vi "update table.vi"(5 "Sort By...":T4 items=["RIO device", "resource", "input type", "datatype", "reserver"], 8 "error in (no error)":errorcluster, 10 "MulticolumnListbox in":refnum<vi>, 11 "Item Ref in":T1 format="%.0x") -> (0 "error out":errorcluster, 2 "max string length in columns":i32[](array[numeric]), 3 "fpga resources out":cluster{"fpga cd":T1, "resource":T2}[](array[cluster]) {"fpga cd" format="%.0x"})   [LabVIEW 2016, in "FPGA RM System Definition API.lvlib"]
uses:
  FPGA RM System Definition API.lvlib
  type defs/viz_type.ctl
  <vilib>/NI Veristand/Custom Device API/Custom Device Item Ref.ctl
  Shared/Types/fpga resource.ctl
  Shared/Types/Channel Type.ctl
  UI/visualizer globals.vi
  <vilib>/NI VeriStand/Custom Device API/Custom Device API.lvlib
  Shared/FPGA RM Shared API.lvlib
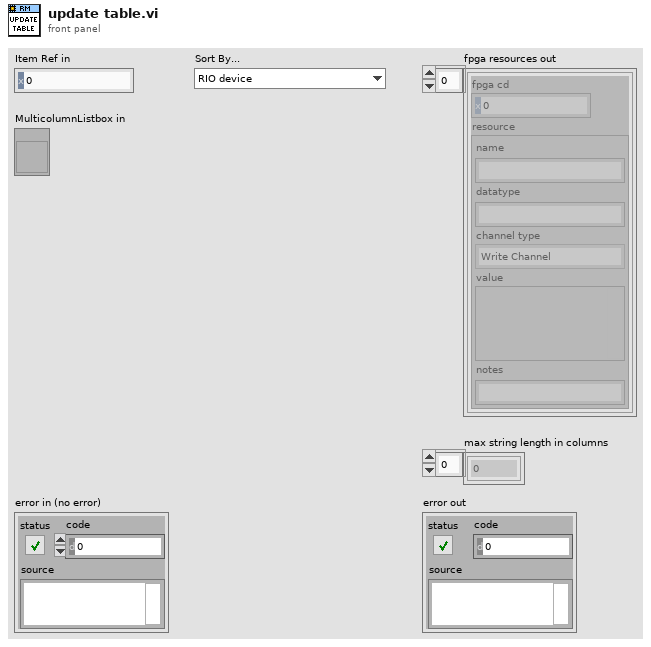
[diagram p1: front panel]
types:
  T1 = typedef "Custom Device API.lvlib/Custom Device Item Ref.ctl" = u64
  T2 = typedef "FPGA RM Shared API.lvlib/fpga resource.ctl" = cluster{"name":string, "datatype":string, "channel type":T3, "value":variant, "notes":string}
  T3 = typedef "FPGA RM Shared API.lvlib/Channel Type.ctl" = enum16{"Write Channel", "Read Channel", "Write Waveform", "Read Waveform"}
  T4 = typedef "FPGA RM System Definition API.lvlib/viz_type.ctl" = u16
  T5 = typedef "FPGA RM System Definition API.lvlib/resources.ctl" = cluster{"fpga cd":T1, "resource":T2}
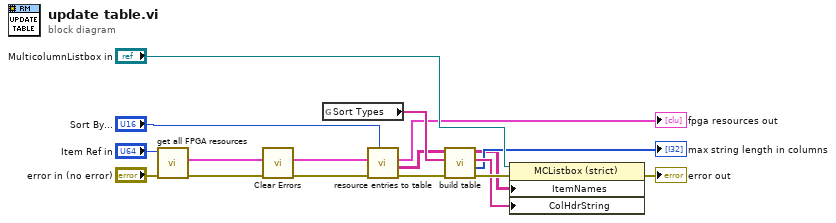
[diagram p0: block diagram]
diagram:
  n1 = call "get all FPGA resources.vi"("error in (no error)"="error in (no error)", "Item Ref in"="Item Ref in") -> ("error out"=w4:errorcluster, "fpga resources"=w3:T5[])  [unwired: 7 in, 1 out]
  n2 = call <vilib>:"Clear Errors.vi"("error in (no error)"=w4) -> ("error out"=w1:errorcluster)  [unwired: 5 in, 1 out]
  n3 = global read "visualizer globals.vi" "Sort Types"() -> (w15:string[])
  n4 = call "resource entries to table.vi"("Sort Type"="Sort By...", "error in (no error)"=w1, "fpga resources"=w3) -> ("error out"=w6:errorcluster, "sorted resource table out"=w10:string[][], "fpga resources"=→"fpga resources out":cluster{"fpga cd":T1, "resource":T2}[])  [unwired: 6 in]
  n5 = call "build table.vi"("error in (no error)"=w6, "Sort Types"=w15, "resource table in"=w10) -> ("error out"=w16:errorcluster, "max string length in columns"=→"max string length in columns":i32[], "Headers"=w14:string[], "resource table out"=w7:string[][])  [unwired: 5 in]
  n6 = property on="Property Node" class="MCListbox (strict)"(reference="MulticolumnListbox in", error in=w16, "ItemNames"=w7, "ColHdrString"=w14) -> (error out=→"error out":errorcluster)  [unwired: 1 out]
